vi "Legend0003.vi"   [LabVIEW 2013]
uses:
  <vilib>/Heliosphere Research LLC/Advanced Plotting Toolkit/api_core/NewPlotType.ctl
  <vilib>/Heliosphere Research LLC/Advanced Plotting Toolkit/api_plotting/Histogram_Automatic.vi
  <vilib>/Heliosphere Research LLC/Advanced Plotting Toolkit/Advanced Plotting Toolkit.lvlib
types:
  T1 = typedef "Advanced Plotting Toolkit.lvlib/NewPlotType.ctl" = enum16{"Rectangular Axes", "Polar Axes"}
  T2 = typedef "Advanced Plotting Toolkit.lvlib/PlotID.ctl" = i32
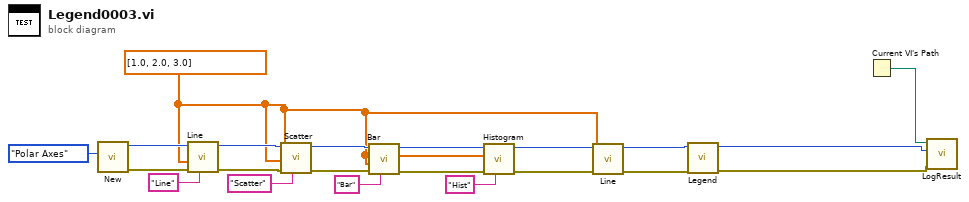
[diagram p0: block diagram]
diagram:
  w2 = dbl[] [1.0, 2.0, 3.0] ("Y Data")
  n1 = call <vilib>:"New.vi"("Plot Type"=NewPlotType."Polar Axes") -> ("error out"=w16:errorcluster, "Plot ID"=w20:T2)  [unwired: 9 in]
  n2 = call <vilib>:"Line.vi"("Legend Title"="Line", "error in (no error)"=w16, "Y Data"=w2, "Plot ID"=w20) -> ("error out"=w15:errorcluster, "Plot ID out"=w19:T2)  [unwired: 6 in]
  n3 = call <vilib>:"Scatter.vi"("Legend Title"="Scatter", "error in (no error)"=w15, "Y Data"=w2, "X Data"=w2, "Plot ID"=w19) -> ("error out"=w14:errorcluster, "Plot ID Out"=w18:T2)  [unwired: 5 in]
  n4 = call <vilib>:"Bar.vi"("Legend Title"="Bar", "error in (no error)"=w14, "Bar Lengths"=w2, "Plot ID"=w18) -> ("error out"=w13:errorcluster, "Plot ID Out"=w17:T2)  [unwired: 6 in]
  n5 = call-poly <vilib>:"Histogram.vi"("Legend Title"="Hist", "error in (no error)"=w13, "Data"=w2, "Plot ID"=w17) -> ("error out"=w5:errorcluster, "Plot ID Out"=w8:T2)  [unwired: 6 in]
  n6 = call <vilib>:"Line.vi"("error in (no error)"=w5, "Y Data"=w2, "Plot ID"=w8) -> ("error out"=w4:errorcluster, "Plot ID out"=w7:T2)  [unwired: 7 in]
  n7 = call <vilib>:"Legend.vi"("error in (no error)"=w4, "Plot ID"=w7) -> ("error out"=w3:errorcluster, "Plot ID Out"=w6:T2)  [unwired: 8 in]
  n8 = Current VI's Path() -> (path=w21:path)
  n9 = call "LogResult.vi"("Test Result"=w3, "Test Artifact"=w6, "VI Path"=w21) -> ()  [unwired: 9 in]
